vi "Calculate AutoSteer and AutoDrive Values.vi"(9 "Distance to Next \nDestination (ft)":dbl, 10 "CW(-1)/CCW(1)":dbl, 11 "Angle to \nNext Destination":dbl) -> (2 "Auto Drive":string, 3 "Auto Steer":string)   [LabVIEW 2011]
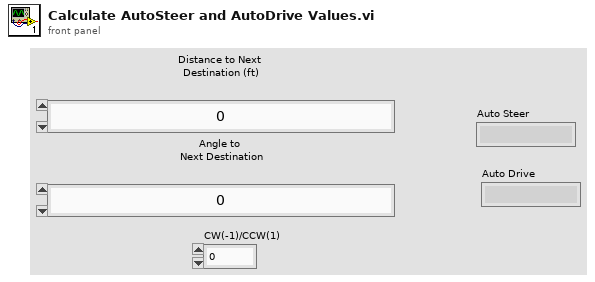
[diagram p1: front panel]
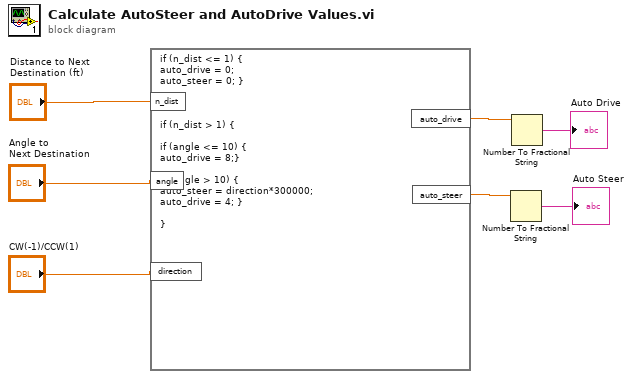
[diagram p0: block diagram]
diagram:
  n1 = formula code="if (n_dist <= 1) {\nauto_drive = 0;\nauto_steer = 0; }\n\n\n\nif (n_dist > 1) {\n\nif (angle <= 10) {\nauto_drive = 8;}\n\nif (angle > 10) {\nauto_steer = direction*300000;\nauto_drive = 4; }\n\n}"("n_dist"="Distance to Next \nDestination (ft)", "angle"="Angle to \nNext Destination", "direction"="CW(-1)/CCW(1)") -> ("auto_drive"=w5:dbl, "auto_steer"=w4:dbl)
  n2 = Number To Fractional String(number=w4) -> (F-format string=→"Auto Steer":string)  [unwired: 3 in]
  n3 = Number To Fractional String(number=w5) -> (F-format string=→"Auto Drive":string)  [unwired: 3 in]
